vi "generatetrianglewaveform.vi"() -> (0 "Waveform":waveform(dbl))   [LabVIEW 2015]
uses:
  <vilib>/measure/NI_MABase.lvlib
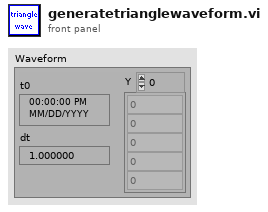
[diagram p1: front panel]
types:
  T1 = cluster{"AO parameters":cluster{"Build analog waveform tabs":dbl, "Repeats":dbl, "Cycles":dbl, "Start amplitude (V)":dbl, "Baseline (V)":dbl, "Step size (V)":dbl, "DC (%)":dbl, "Sampling frequency (Hz)":dbl, "Period (ms)":dbl, "Offset (V)":dbl, "Amplitude (V)":dbl, "Frequency":dbl, "Tri Repeats":dbl, "Cycle length (s)":dbl, "Pulses":dbl, "Matlab wave number":dbl}[], "DO parameters":cluster{"Digital DC (%)":dbl, "Digital phase":dbl, "Digital Freq (Hz)":dbl, "Sampling frequency (Hz)":dbl}[]}
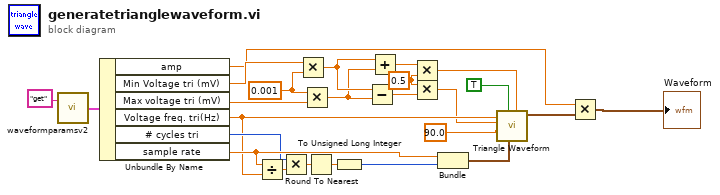
[diagram p0: block diagram]
diagram:
  w11 = 0.001
  w6 = 0.5 ("y")
  n1 = call "waveformparamsv2.vi"("command"="get") -> ("Params out"=w21:T1)  [unwired: 1 in]
  n2 = Unbundle By Name(w21) -> ("amp"=w2:dbl, "Min Voltage tri (mV)"=w10:dbl, "Max voltage tri (mV)"=w12:dbl, "Voltage freq. tri(Hz)"=w17:dbl, "# cycles tri"=w18:u32, "sample rate"=w20:dbl)
  n3 = Divide(x=w20, y=w17) -> (x/y=w19:dbl)
  n4 = Multiply(x=w18, y=w19) -> (x*y=w25:dbl)
  n5 = Multiply(x=w10, y=w11) -> (x*y=w9:dbl)
  n6 = Multiply(x=w11, y=w12) -> (x*y=w8:dbl)
  n7 = Round To Nearest(number=w25) -> (nearest integer value=w24:dbl)
  n8 = To Unsigned Long Integer(number=w24) -> (unsigned 32bit integer=w23:u32)
  n9 = Subtract(x=w9, y=w8) -> (x-y=w5:dbl)
  n10 = Add(x=w9, y=w8) -> (x+y=w7:dbl)
  n11 = Multiply(x=w7, y=w6) -> (x*y=w4:dbl)
  n12 = Multiply(x=w6, y=w5) -> (x*y=w3:dbl)
  n13 = Bundle("sample rate"=w20, w23) -> (w15:cluster{"sample rate":dbl, u32})  [unwired: 1 out]
  n14 = call <vilib>:"Triangle Waveform.vi"("offset"=w4, "sampling info"=w15, "reset signal"=TRUE, "phase"=90.0, "amplitude"=w3, "frequency"=w17) -> ("signal out"=w13:waveform(dbl))  [unwired: 4 in, 1 out]
  n15 = Multiply(x=w2, y=w13) -> (x*y=→"Waveform":waveform(dbl))
